vi "write_tags_subvi.vi"(0 "NI Skyline Tag in":refnum<class "NI Skyline Tag.lvclass">, 1 "Warn String":refnum<class "NI Skyline Tag.lvclass">, 2 "Warmer\nON":bool, 3 "HOT\nSurface":bool, 5 "Coffee-T":refnum<class "NI Skyline Tag.lvclass">, 7 "Plate-T":refnum<class "NI Skyline Tag.lvclass">, 9 "Hot-Sfc":refnum<class "NI Skyline Tag.lvclass">, 12 "Numeric":dbl, 13 "String":string, 14 "Numeric 2":dbl) -> (4 "NI Skyline Tag out":refnum<class "NI Skyline Tag.lvclass">, 6 "tag out 4":refnum<class "NI Skyline Tag.lvclass">, 8 "tag out 3":refnum<class "NI Skyline Tag.lvclass">, 10 "tag out 2":refnum<class "NI Skyline Tag.lvclass">, 15 "tag out":refnum<class "NI Skyline Tag.lvclass">)   [LabVIEW 2021]
uses:
  <vilib>/Skyline/Tag/Wrapper/Wrapper_class/NI Skyline Tag.lvclass
  <vilib>/Skyline/Tag/Wrapper/Wrapper_class/Write Tag (DBL).vi
  <vilib>/Skyline/Tag/Wrapper/Wrapper_class/Write Tag (Boolean).vi
  <vilib>/Skyline/Tag/Wrapper/Wrapper_class/Write Tag (String).vi
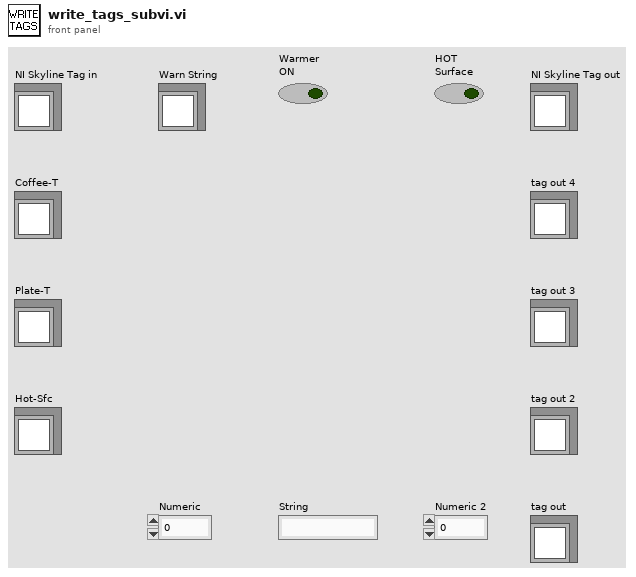
[diagram p1: front panel]
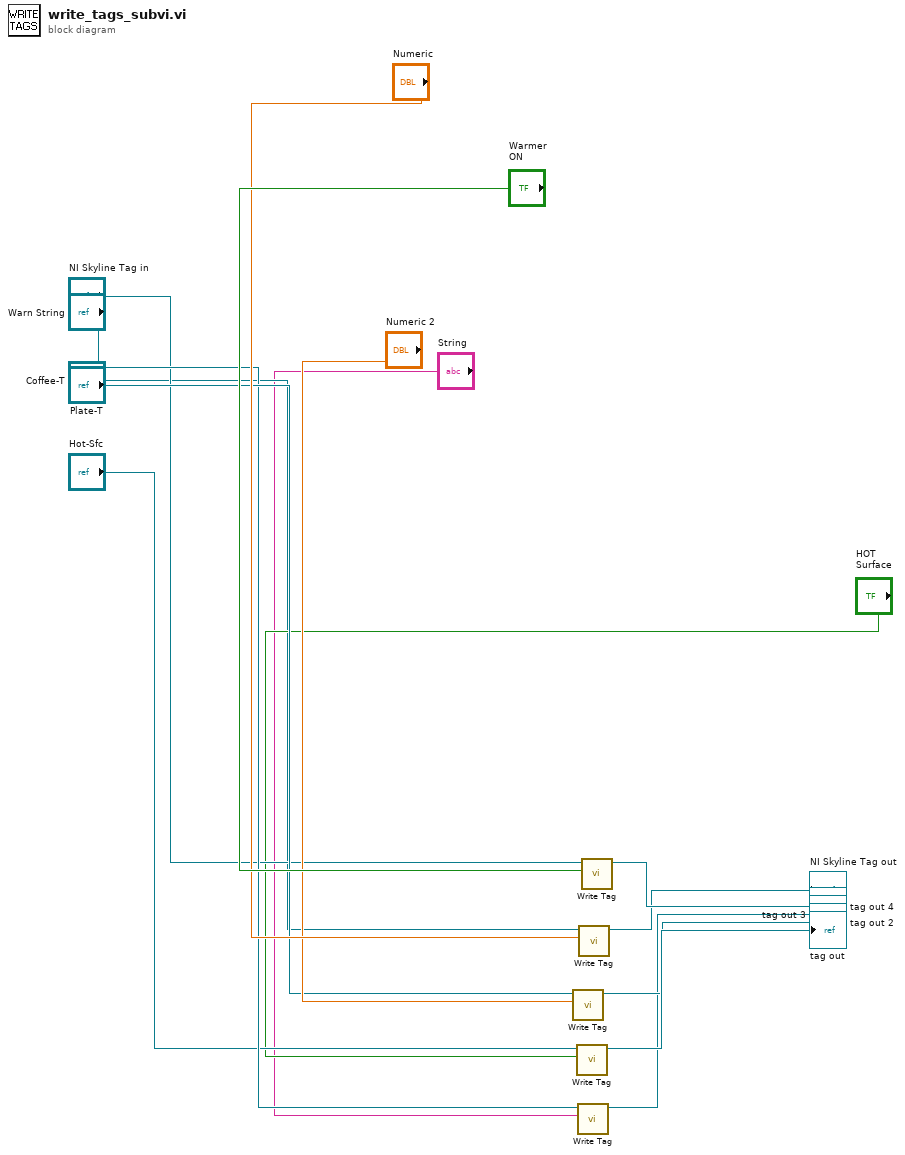
[diagram p0: block diagram]
diagram:
  n1 = call-poly <vilib>:"Write Tag.vi"("value"="Numeric 2", "tag in"="Plate-T") -> ("tag out"=→"tag out 2":refnum<class "NI Skyline Tag.lvclass">)  [unwired: 8 in, 1 out]
  n2 = call-poly <vilib>:"Write Tag.vi"("value"="HOT\nSurface", "tag in"="Hot-Sfc") -> ("tag out"=→"tag out":refnum<class "NI Skyline Tag.lvclass">)  [unwired: 8 in, 1 out]
  n3 = call-poly <vilib>:"Write Tag.vi"("value"="String", "tag in"="Warn String") -> ("tag out"=→"tag out 3":refnum<class "NI Skyline Tag.lvclass">)  [unwired: 8 in, 1 out]
  n4 = call-poly <vilib>:"Write Tag.vi"("value"="Numeric", "tag in"="Coffee-T") -> ("tag out"=→"NI Skyline Tag out":refnum<class "NI Skyline Tag.lvclass">)  [unwired: 8 in, 1 out]
  n5 = call-poly <vilib>:"Write Tag.vi"("value"="Warmer\nON", "tag in"="NI Skyline Tag in") -> ("tag out"=→"tag out 4":refnum<class "NI Skyline Tag.lvclass">)  [unwired: 8 in, 1 out]
